vi "Configure Analog Gen Noise.vi"(0 "VISA resource name":refnum<visa-resource-name>, 1 "Enable Repeat Period (T: Enable)":bool=TRUE, 2 "Enable Waveform (T: Enable)":bool=TRUE, 3 "Filter Type (0: nsNoFilter)":i32(ring) items=["nsNoFilter", "nsLoPass", "nsHiPass", "nsBandPassOct3"], 5 "Channel (0: A)":i32(ring) items=["A", "B"], 9 "Noise Amplitude (0 Vrms)":dbl, 11 "error in (no error)":errorcluster, 12 "Enable Pinking Filter (T: Enable)":bool=TRUE, 13 "Repeat Period (0.01 s)":dbl=0.01, 14 "Filter Frequency (10 Hz)":dbl=10.0) -> (4 "VISA resource name out":refnum<visa-resource-name>, 15 "error out":errorcluster)   [LabVIEW 2014, in "Stanford Research SR1.lvlib"]
doc: "Configures the attributes for the Analog Generator Noise."
uses:
  Stanford Research SR1.lvlib
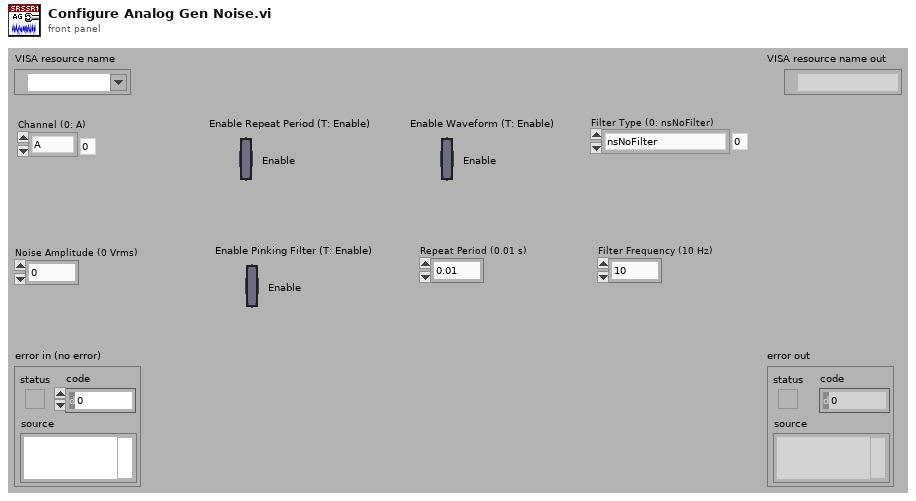
[diagram p1: front panel]
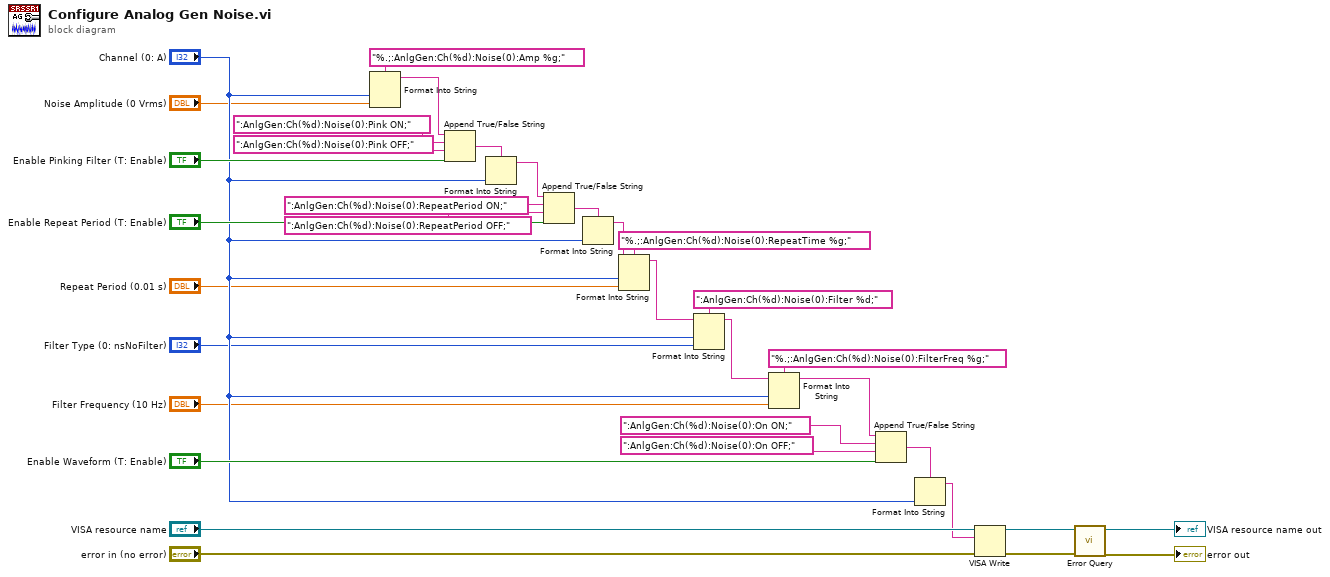
[diagram p0: block diagram]
diagram:
  n1 = Format Into String(format string="%.;:AnlgGen:Ch(%d):Noise(0):Amp %g;", "Channel (0: A)", "Noise Amplitude (0 Vrms)") -> (resulting string=w33:string)  [unwired: 2 in, 1 out]
  n2 = Append True/False String(1:"Enable Pinking Filter (T: Enable)", 2:":AnlgGen:Ch(%d):Noise(0):Pink OFF;", 3:":AnlgGen:Ch(%d):Noise(0):Pink ON;", 4:w33) -> (0:w11:string)
  n3 = Format Into String(format string=w11, "Channel (0: A)") -> (resulting string=w10:string)  [unwired: 2 in, 1 out]
  n4 = Append True/False String(1:"Enable Repeat Period (T: Enable)", 2:":AnlgGen:Ch(%d):Noise(0):RepeatPeriod OFF;", 3:":AnlgGen:Ch(%d):Noise(0):RepeatPeriod ON;", 4:w10) -> (0:w13:string)
  n5 = Format Into String(format string=w13, "Channel (0: A)") -> (resulting string=w12:string)  [unwired: 2 in, 1 out]
  n6 = Format Into String(format string="%.;:AnlgGen:Ch(%d):Noise(0):RepeatTime %g;", initial string=w12, "Channel (0: A)", "Repeat Period (0.01 s)") -> (resulting string=w25:string)  [unwired: 1 in, 1 out]
  n7 = Format Into String(format string=":AnlgGen:Ch(%d):Noise(0):Filter %d;", initial string=w25, "Channel (0: A)", "Filter Type (0: nsNoFilter)") -> (resulting string=w23:string)  [unwired: 1 in, 1 out]
  n8 = Format Into String(format string="%.;:AnlgGen:Ch(%d):Noise(0):FilterFreq %g;", initial string=w23, "Channel (0: A)", "Filter Frequency (10 Hz)") -> (resulting string=w8:string)  [unwired: 1 in, 1 out]
  n9 = Append True/False String(1:"Enable Waveform (T: Enable)", 2:":AnlgGen:Ch(%d):Noise(0):On OFF;", 3:":AnlgGen:Ch(%d):Noise(0):On ON;", 4:w8) -> (0:w7:string)
  n10 = Format Into String(format string=w7, "Channel (0: A)") -> (resulting string=w6:string)  [unwired: 2 in, 1 out]
  n11 = VISA Write(VISA resource name="VISA resource name", write buffer=w6, error in (no error)="error in (no error)") -> (VISA resource name out=w17:refnum<visa-resource-name>, error out=w16:errorcluster)  [unwired: 1 out]
  n12 = call "Error Query.vi"("error in (no error)"=w16, "VISA resource name"=w17) -> ("error out"=→"error out":errorcluster, "VISA resource name out"=→"VISA resource name out":refnum<visa-resource-name>)  [unwired: 6 in, 2 out]
